vi "Get Descriptor.vi"(11 "output_actor in":refnum<class "test_hardwareactor.lvclass">) -> (2 "Descriptor":string, 3 "output_actor out":refnum<class "test_hardwareactor.lvclass">)   [LabVIEW 2015, in "test_hardwareactor.lvclass"]
uses:
  test_hardwareactor.lvclass
  Output Actor Hardware/Output Actor Hardware.lvclass
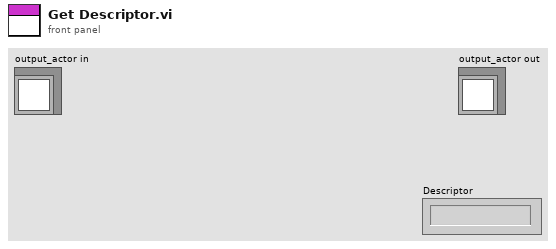
[diagram p1: front panel]
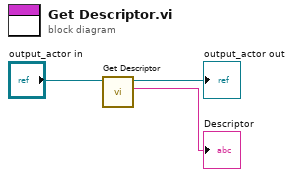
[diagram p0: block diagram]
diagram:
  n1 = call-parent "Get Descriptor.vi"("output_actor in"="output_actor in") -> ("Descriptor"=→"Descriptor":string, "output_actor out"=→"output_actor out":refnum<class "test_hardwareactor.lvclass">)  [unwired: 9 in]
